vi "Write Byte.vi"(7 "1-Wire DIO Pin":refnum<k21>="ConnectorA/DIO15", 8 "error in":errorcluster, 10 "Tx data":u8) -> (0 "error out":errorcluster)   [LabVIEW 2014, in "Maxim 1-Wire.lvlib"]
doc: "Writes a byte stored in a U8 to the 1-Wire bus."
uses:
  Maxim 1-Wire.lvlib
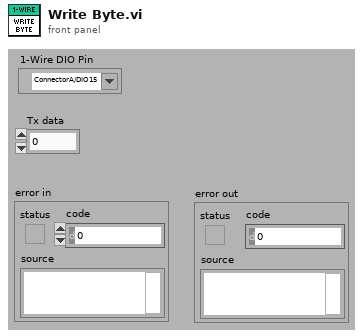
[diagram p1: front panel]
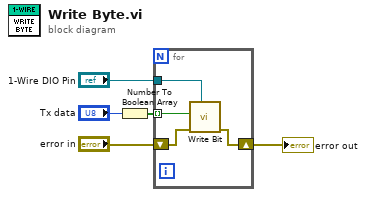
[diagram p0: block diagram]
diagram:
  n1 = Number To Boolean Array(number="Tx data") -> (Boolean array=w5:bool[])
  n2 = for {
    tunnel: w5 -> [w8] mode=indexing
    tunnel: "1-Wire DIO Pin" -> [w9]
    shift-right: [w6] -> w1
    shift-left: "error in" -> [w7]
    n3 = call "Write Bit.vi"("1-Wire DIO Pin"=w9, "Error In"=w7, "Bit"=w8) -> ("Error Out"=w6:errorcluster)  [unwired: 8 in]
  }
  "error out" <- w1
